vi "Level1ClassGetter.vi"(8 "error in (no error)":errorcluster, 11 "ALevel2ClassCopy in":refnum<class "ALevel2ClassCopy.lvclass">) -> (0 "error out":errorcluster, 1 "Level1Class out":refnum<class "Level1Class.lvclass">, 3 "ALevel2ClassCopy out":refnum<class "ALevel2ClassCopy.lvclass">)   [LabVIEW 2019, in "ALevel2ClassCopy.lvlib" / "ALevel2ClassCopy.lvclass"]
uses:
  ALevel2ClassCopy.lvclass
  Level1Class/Level1Class.lvclass
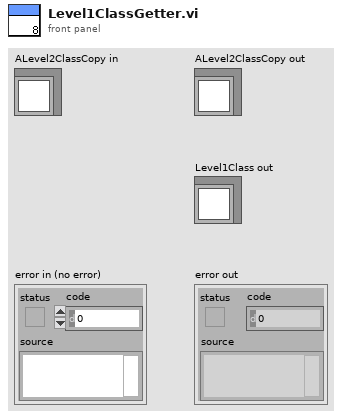
[diagram p1: front panel]
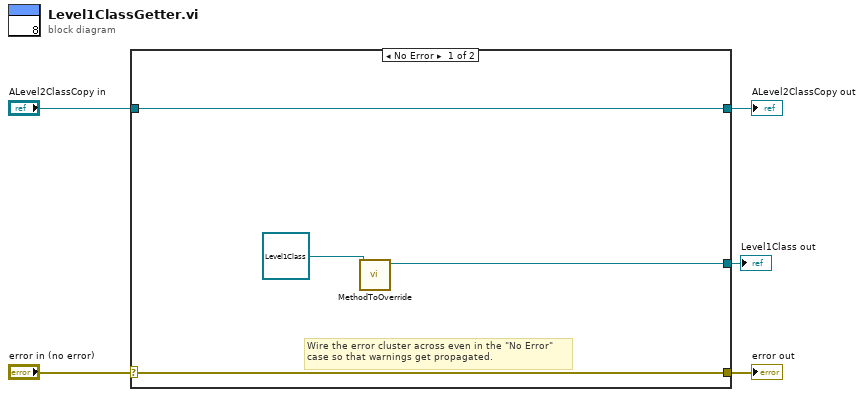
[diagram p0: block diagram]
diagram:
  n1 = case shown="No Error" "error in (no error)" {
    selector: "error in (no error)" -> [w8 w11]
    tunnel: [w8 w11] -> w4
    tunnel: [w9 w10] -> w2
    tunnel: "ALevel2ClassCopy in" -> [w9 w10]
    tunnel: [w6 _] -> w1
    frame No Error {
      # "Wire the error cluster across even in the \"No Error\"\ncase so that warnings get propagated."
      n2 = call-dynamic "MethodToOverride.vi"("Level1Class in"=refnum<class "Level1Class.lvclass"> refnum ("Level1Class.lvlib:Level1Class.lvclass")) -> ("Level1Class out"=w6:refnum<class "Level1Class.lvclass">)  [unwired: 9 in, 1 out]
    }
    frame Error {
    }
  }
  "error out" <- w4
  "ALevel2ClassCopy out" <- w2
  "Level1Class out" <- w1
